vi "CreateMazeOLD.vi"(8 "error in (no error)":errorcluster, 11 "MazeGame in":refnum<class "MazeGame.lvclass">) -> (0 "error out":errorcluster, 2 "Maze":refnum<class "Maze.lvclass">, 3 "MazeGame out":refnum<class "MazeGame.lvclass">)   [LabVIEW 2020, in "FactoryMethod.lvlib" / "NoParametrizedFactoryMethod.lvlib" / "MazeGame.lvclass"]
uses:
  MazeGame.lvclass
  GoFcommonClasses/Maze/Maze.lvclass
  GoFcommonClasses/Direction.ctl
  Private/TypeDef/RoomElement.ctl
  GoFcommonClasses/MazeSite/MazeSite.lvclass
  GoFcommonClasses/ConcreteMazeSite/Door/Door.lvclass
  E:/GitHub/Design-Patterns-GoF_-_NI-LV/Creational/GoFcommonClasses/MazeSite/MazeSite.lvclass
  GoFcommonClasses/ConcreteMazeSite/Room/Room.lvclass
  Support/Class/ConsoleOutput.lvclass
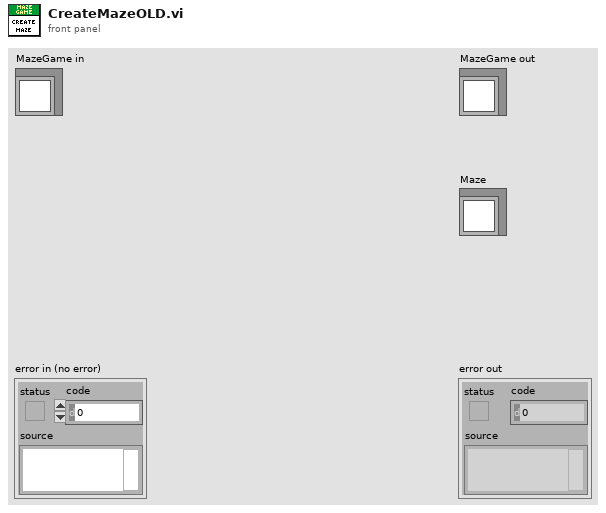
[diagram p1: front panel]
types:
  T1 = typedef "Room.lvclass/RoomElement.ctl" = cluster{"Direction":T2, "MazeSite":refnum<class "MazeSite.lvclass">}
  T2 = typedef "Direction.ctl" = enum32{"North", "South", "East", "West"}
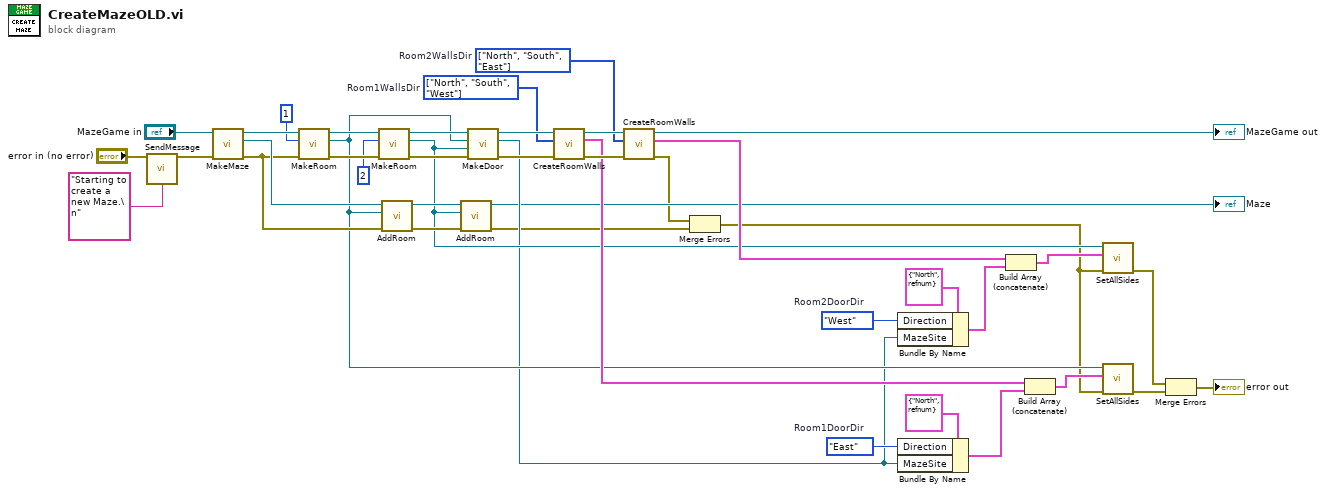
[diagram p0: block diagram]
diagram:
  w37 = Direction."West"  # Room2DoorDir
  w38 = Direction."East"  # Room1DoorDir
  w10 = T2[] [enum."North", enum."South", enum."East"] items=["North", "South", "East", "West"]  # Room2WallsDir
  w11 = T2[] [enum."North", enum."South", enum."West"] items=["North", "South", "East", "West"]  # Room1WallsDir
  n1 = call "SendMessage.vi"("Message"="Starting to create a new Maze.\n", "error in (no error)"="error in (no error)") -> ("error out"=w15:errorcluster)  [unwired: 13 in]
  n2 = call-dynamic "MakeMaze.vi"("error in (no error)"=w15, "MazeGame in"="MazeGame in") -> ("error out"=w14:errorcluster, "Maze"=w16:refnum<class "Maze.lvclass">, "MazeGame out"=w22:refnum<class "MazeGame.lvclass">)  [unwired: 7 in]
  n3 = call-dynamic "MakeRoom.vi"("error in (no error)"=w14, "RoomNumber"=1, "MazeGame in"=w22) -> ("error out"=w23:errorcluster, "Room"=w6:refnum<class "Room.lvclass">, "MazeGame out"=w21:refnum<class "MazeGame.lvclass">)  [unwired: 6 in]
  n4 = call-dynamic "MakeRoom.vi"("error in (no error)"=w23, "RoomNumber"=2, "MazeGame in"=w21) -> ("error out"=w18:errorcluster, "Room"=w7:refnum<class "Room.lvclass">, "MazeGame out"=w17:refnum<class "MazeGame.lvclass">)  [unwired: 6 in]
  n5 = call "AddRoom.vi"("error in (no error)"=w14, "Room"=w6, "Maze in"=w16) -> ("error out"=w41:errorcluster, "Maze out"=w40:refnum<class "Maze.lvclass">)  [unwired: 7 in]
  n6 = call "AddRoom.vi"("error in (no error)"=w41, "Room"=w7, "Maze in"=w40) -> ("error out"=w3:errorcluster, "Maze out"=→"Maze":refnum<class "Maze.lvclass">)  [unwired: 7 in]
  n7 = call-dynamic "MakeDoor.vi"("error in (no error)"=w18, "Room 2"=w7, "Room 1"=w6, "MazeGame in"=w17) -> ("error out"=w13:errorcluster, "Door"=w5:refnum<class "Door.lvclass">, "MazeGame out"=w12:refnum<class "MazeGame.lvclass">)  [unwired: 5 in]
  n8 = call "CreateRoomWalls.vi"("error in (no error)"=w13, "DirectionsList"=w11, "MazeGame in"=w12) -> ("error out"=w28:errorcluster, "RoomWallsList"=w8:T1[], "MazeGame out"=w27:refnum<class "MazeGame.lvclass">)  [unwired: 6 in]
  n9 = call "CreateRoomWalls.vi"("error in (no error)"=w28, "DirectionsList"=w10, "MazeGame in"=w27) -> ("error out"=w2:errorcluster, "RoomWallsList"=w9:T1[], "MazeGame out"=→"MazeGame out":refnum<class "MazeGame.lvclass">)  [unwired: 6 in]
  n10 = Merge Errors(w2, w3) -> (w1:errorcluster)
  n11 = Bundle By Name(cluster=T1 {"Direction"=enum."North", "MazeSite"=refnum} ("RoomElement"), "Direction"=w37, "MazeSite"=w5) -> (w34:T1)
  n12 = Bundle By Name(cluster=T1 {"Direction"=enum."North", "MazeSite"=refnum} ("RoomElement"), "Direction"=w38, "MazeSite"=w5) -> (w35:T1)
  n13 = Build Array (concatenate)(w9, w34) -> (w26:T1[])
  n14 = Build Array (concatenate)(w8, w35) -> (w25:T1[])
  n15 = call "SetAllSides.vi"("error in (no error)"=w1, "RoomSides"=w26, "Room in"=w7) -> ("error out"=w33:errorcluster)  [unwired: 7 in, 1 out]
  n16 = call "SetAllSides.vi"("error in (no error)"=w1, "RoomSides"=w25, "Room in"=w6) -> ("error out"=w32:errorcluster)  [unwired: 7 in, 1 out]
  n17 = Merge Errors(w33, w32) -> (→"error out":errorcluster)
